vi "Create Pulse Waveform.vi"(8 "error in (no error)":errorcluster, 11 "Waveform parameters":T1={"Sample rate"=6389760000.0, "Carrier frequency"=217000000.0, "Carrier amplitude"=217000000.0, "Number of waves"=75.0, "Standard deviation"=0.1, "Add trigger wfrm"=TRUE, "Waveform pattern"=enum."Only signal"} {"Carrier amplitude" format="%#_6p"; "Standard deviation" format="%#_6p"; "Number of waves" format="%#_6p"; "Carrier frequency" format="%#_6pHz"; "Sample rate" format="%#_6pHz"}) -> (0 "error out":errorcluster, 1 "Trigger":dbl[](array[numeric]), 2 "Signal":dbl[](array[numeric]))   [LabVIEW 2024]
uses:
  Pulse Waveform Parameters.ctl
  <vilib>/Analysis/4window.llb/Gaussian Window (DBL).vi
  <vilib>/Analysis/NI_AALPro.lvlib
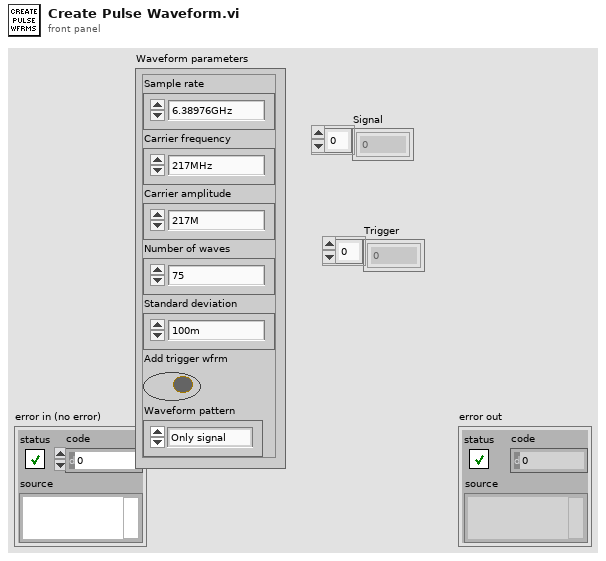
[diagram p1: front panel]
types:
  T1 = typedef "Pulse Waveform Parameters.ctl" = cluster{"Sample rate":dbl, "Carrier frequency":dbl, "Carrier amplitude":dbl, "Number of waves":dbl, "Standard deviation":dbl, "Add trigger wfrm":bool, "Waveform pattern":enum16{"Only signal", "Sig + Trig", "Two triggers"}}
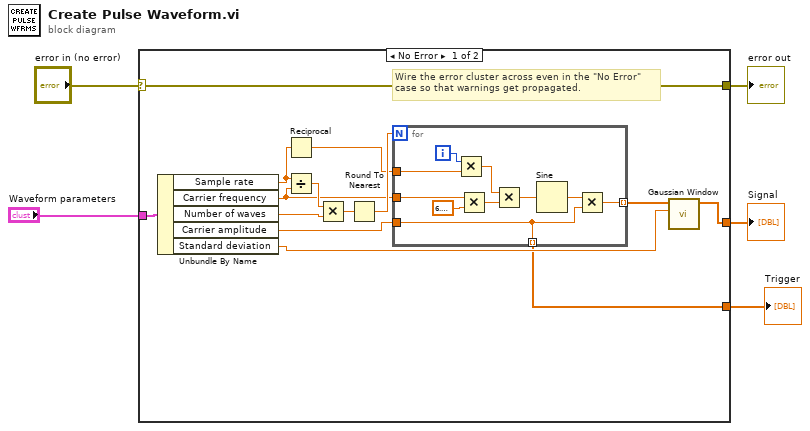
[diagram p0: block diagram]
diagram:
  n1 = case shown="No Error" "error in (no error)" {
    selector: "error in (no error)" -> [w15 w30]
    tunnel: [w15 w30] -> w4
    tunnel: [w13 _] -> w3
    tunnel: "Waveform parameters" -> [w12 _]
    tunnel: [w6 _] -> w1
    frame No Error {
      # "Wire the error cluster across even in the \"No Error\"\ncase so that warnings get propagated."
      n2 = Unbundle By Name(w12) -> ("Sample rate"=w11:dbl, "Carrier frequency"=w10:dbl, "Number of waves"=w8:dbl, "Carrier amplitude"=w9:dbl, "Standard deviation"=w7:dbl)
      n3 = Reciprocal(x=w11) -> (1/x=w16:dbl)
      n4 = Divide(x=w11, y=w10) -> (x/y=w19:dbl)
      n5 = Multiply(x=w19, y=w8) -> (x*y=w18:dbl)
      n6 = Round To Nearest(number=w18) -> (nearest integer value=w17:dbl)
      n7 = for {
        N: w17 -> [_]
        tunnel: [w24] -> w14 mode=indexing
        tunnel: w10 -> [w21]
        tunnel: w16 -> [w22]
        tunnel: w9 -> [w20]
        tunnel: [w20] -> w6 mode=indexing
        i -> [w23]
        n8 = Multiply(x=w23, y=w22) -> (x*y=w26:dbl)
        n9 = Multiply(x=w21, y=6.283185307179586) -> (x*y=w27:dbl)
        n10 = Multiply(x=w26, y=w27) -> (x*y=w29:dbl)
        n11 = Sine(x=w29) -> (sin(x)=w25:dbl)
        n12 = Multiply(x=w25, y=w20) -> (x*y=w24:dbl)
      }
      n13 = call-poly <vilib>:"Gaussian Window.vi"("standard deviation"=w7, "X"=w14) -> ("Windowed X"=w13:dbl[])  [unwired: 8 in, 1 out]
    }
    frame Error {
    }
  }
  "error out" <- w4
  "Signal" <- w3
  "Trigger" <- w1
